vi "HostToFPGA(RGB).vi"(7 "Maximum Pixels per Write":i32=-1, 8 "error in (no error)":errorcluster, 9 "FPGA Reference in":refnum<k20>, 10 "Write Timeout (ms)":i32=5000, 11 "Image in":T1) -> (0 "error out":errorcluster, 3 "Image out":T1)   [LabVIEW 2016]
uses:
  <vilib>/vision/Image Controls.llb/IMAQ Image.ctl
  <vilib>/vision/EDVR.llb/IMAQ ImageToEDVR 2D U32.vi
  <vilib>/rvi/errors/niLvFpgaAdjustHostInterfaceError.vi
  <vilib>/rvi/interface/nirviMethod/nirviMethod.xnode
  <vilib>/FPGAPlugInAG/Dynamic/niLvFpga_WriteFifo_Dynamic.vi
  <vilib>/rvi/errors/niLvFpgaMergeErrorWithErrorCode.vi
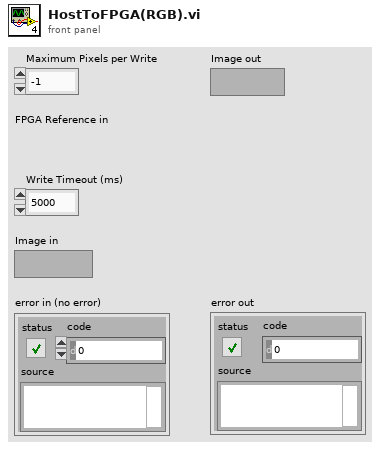
[diagram p1: front panel]
types:
  T1 = typedef "IMAQ Image.ctl" = refnum<image>
  T2 = typedef "Image Type" = u32
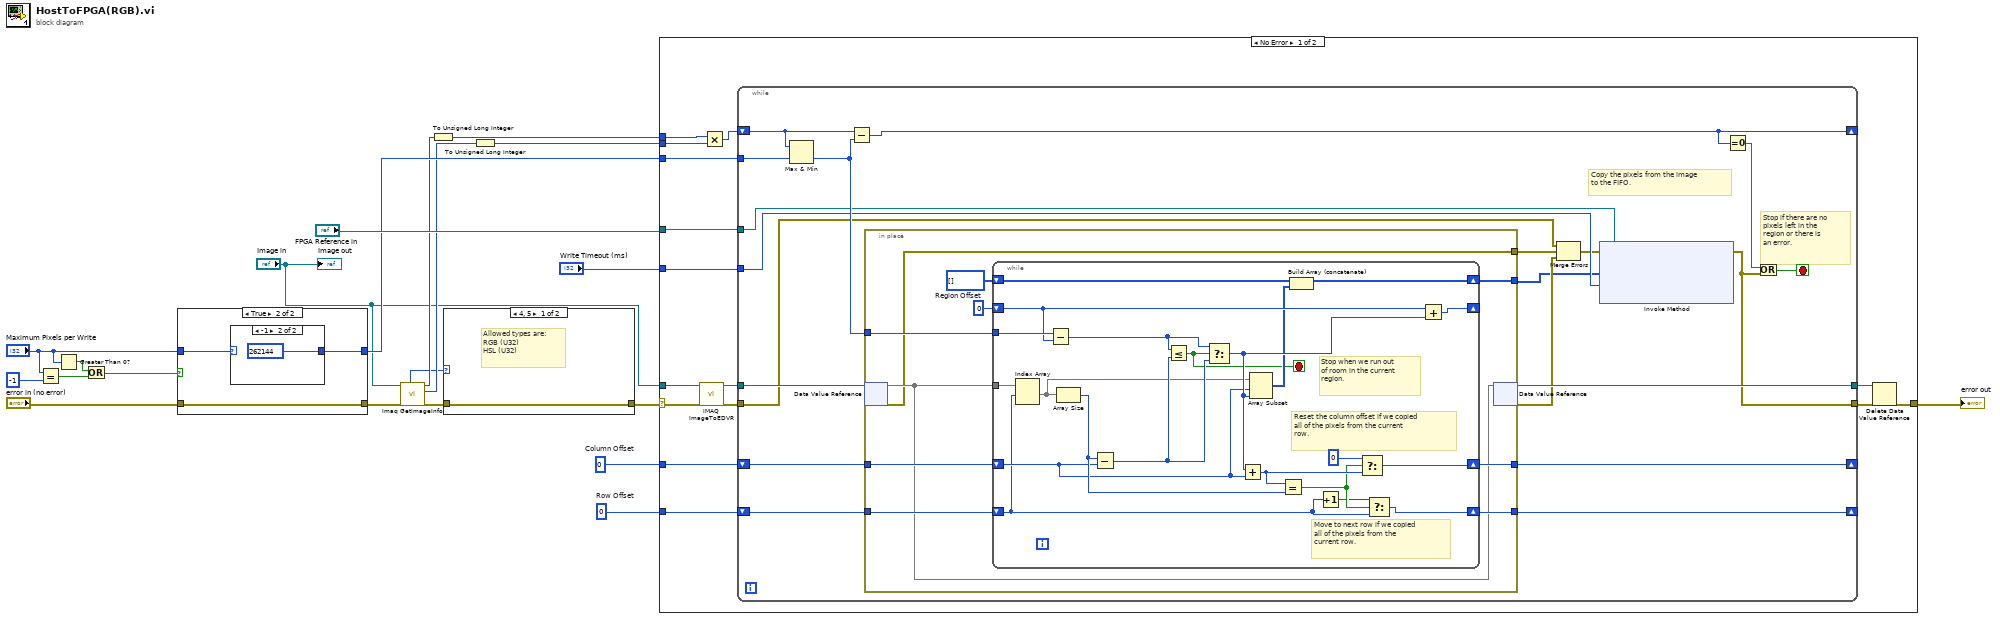
[diagram p0: block diagram]
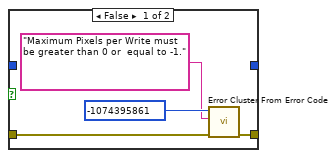
[diagram p2: hidden frame]
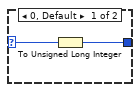
[diagram p3: hidden frame]
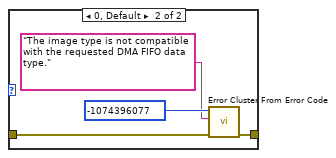
[diagram p4: hidden frame]
diagram:
  w14 = u32 0  # Row Offset
  w15 = u32 0  # Column Offset
  n1 = Equal?(x="Maximum Pixels per Write", y=-1) -> (x = y?=w5:bool)
  n2 = Greater Than 0?(x="Maximum Pixels per Write") -> (x > 0?=w4:bool)
  n3 = Or(x=w4, y=w5) -> (x .or. y?=w6:bool)
  n4 = case shown="True" w6 {
    tunnel: "error in (no error)" -> [w23 w28]
    tunnel: [w22 w28] -> w12
    tunnel: "Maximum Pixels per Write" -> [_ w27]
    tunnel: [_ w26] -> w18
    frame False {
      n5 = call <vilib>:"Error Cluster From Error Code.vi"("error in (no error)"=w23, "error message (\"\")"="Maximum Pixels per Write must be greater than 0 or  equal to -1." ("error message (\"\")"), "error code (0)"=-1074395861) -> ("error out"=w22:errorcluster)  [unwired: 6 in]
    }
    frame True {
      n6 = case shown="-1" w27 {
        selector: w27 -> [w30 _]
        tunnel: [w29 u32 262144 ("Maximum Pixels per Write")] -> w26
        frame 0, Default {
          n7 = To Unsigned Long Integer(number=w30) -> (unsigned 32bit integer=w29:u32)
        }
        frame -1 {
        }
      }
    }
  }
  n8 = call "Imaq GetImageInfo"("error in (no error)"=w12, "Image"="Image in") -> ("error out"=w11:errorcluster, "Y Resolution"=w17:i32, "X Resolution"=w13:i32, "Image Type"=w10:T2)  [unwired: 2 in, 4 out]
  n9 = To Unsigned Long Integer(number=w13) -> (unsigned 32bit integer=w19:u32)
  n10 = case shown="4, 5" w10 {
    tunnel: w11 -> [w32 w34]
    tunnel: [w32 w33] -> w16
    frame 4, 5 {
      # "Allowed types are:\nRGB (U32)\nHSL (U32)"
    }
    frame 0, Default {
      n11 = call <vilib>:"Error Cluster From Error Code.vi"("error in (no error)"=w34, "error message (\"\")"="The image type is not compatible with the requested DMA FIFO data type." ("error message (\"\")"), "error code (0)"=-1074396077) -> ("error out"=w33:errorcluster)  [unwired: 6 in]
    }
  }
  n12 = To Unsigned Long Integer(number=w17) -> (unsigned 32bit integer=w20:u32)
  n13 = case shown="No Error" w16 {
    selector: w16 -> [w46 w103]
    tunnel: w15 -> [w48 _]
    tunnel: w14 -> [w47 _]
    tunnel: "FPGA Reference in" -> [w50 _]
    tunnel: [w44 w103] -> w8
    tunnel: w18 -> [w51 _]
    tunnel: "Write Timeout (ms)" -> [w49 _]
    tunnel: "Image in" -> [w45 _]
    tunnel: w19 -> [w43 _]
    tunnel: w20 -> [w42 _]
    frame No Error {
      n14 = call-poly <vilib>:"IMAQ ImageToEDVR.vi"("error out"=w46, "Image"=w45) -> ("error out"=w40:errorcluster, "EDVR 2D U32"=w41:refnum<data-value>)  [unwired: 7 in, 1 out]
      n15 = Multiply(x=w43, y=w42) -> (x*y=w37:u32)
      n16 = while {
        shift-right: [w65] -> _
        shift-left: w37 -> [w62]
        tunnel: w41 -> [w71]
        shift-right: [w67] -> _
        shift-left: w48 -> [w69]
        shift-right: [w70] -> _
        shift-left: w47 -> [w68]
        tunnel: w50 -> [w56]
        tunnel: [w66] -> w39
        tunnel: [w54] -> w38
        tunnel: w51 -> [w61]
        tunnel: w49 -> [w57]
        tunnel: w40 -> [w52]
        stop <- w64 stop-if-true
        # "Copy the pixels from the image\nto the FIFO."
        # "Stop if there are no\npixels left in the \nregion or there is\nan error."
        n17 = Max & Min(x=w62, y=w61) -> (min(x,y)=w60:u32)  [unwired: 1 out]
        n18 = Subtract(x=w62, y=w60) -> (x-y=w65:u32)
        n19 = in-place {
          in-place-border: w60 -> [w79]
          in-place-border: [w81] -> w70
          in-place-border: w69 -> [w78]
          in-place-border: w68 -> [w76]
          in-place-border: [w77] -> w67
          in-place-border: [w73] -> w59
          in-place-border: [w72] -> w53
          w80 = u32 0  # Region Offset
          n20 = in-place-dvr #1(w71) -> (w75:u32[][], w73:errorcluster)
          n21 = while {
            tunnel: w75 -> [w88]
            shift-right: [w100] -> _
            shift-left: w80 -> [w99]
            tunnel: w79 -> [w102]
            shift-right: [w93] -> w77
            shift-left: w78 -> [w89]
            shift-right: [w83] -> w72
            shift-left: u8[] [] -> [w85]
            shift-right: [w90] -> w81
            shift-left: w76 -> [w86]
            stop <- w82 stop-if-true
            # "Stop when we run out\nof room in the current\nregion."
            # "Reset the column offset if we copied\nall of the pixels from the current\nrow."
            # "Move to next row if we copied\nall of the pixels from the\ncurrent row."
            n22 = Index Array(array=w88, index (row)=w86) -> (element=w87:u32[])  [unwired: 1 in]
            n23 = Subtract(x=w102, y=w99) -> (x-y=w101:u32)
            n24 = Array Size(array=w87) -> (size(s)=w98:i32)
            n25 = Subtract(x=w98, y=w89) -> (x-y=w96:u32)
            n26 = Less Or Equal?(x=w101, y=w96) -> (x <= y?=w82:bool)
            n27 = Select(t=w101, s=w82, f=w96) -> (s? t:f=w97:u32)
            n28 = Add(x=w97, y=w89) -> (x+y=w94:u32)
            n29 = Array Subset(array=w87, index=w89, length=w97) -> (w84:u32[])
            n30 = Equal?(x=w94, y=w98) -> (x = y?=w92:bool)
            n31 = Build Array (concatenate)(w85, w84) -> (w83:u32[])
            n32 = Increment(x=w86) -> (x+1=w91:u32)
            n33 = Select(t=u32 0 ("Elements In Region"), s=w92, f=w94) -> (s? t:f=w93:u32)
            n34 = Select(t=w91, s=w92, f=w86) -> (s? t:f=w90:u32)
            n35 = Add(x=w99, y=w97) -> (x+y=w100:u32)
          }
          n36 = in-place-dvr #1(w75) -> (w66:refnum<data-value>, w58:errorcluster)
        }
        n37 = Merge Errors(w52, w59, w58) -> (w55:errorcluster)
        n38 = xnode "Invoke Method"("FPGA VI Reference In"=w56, "error in"=w55, "Data"=w53, "Timeout (ms)"=w57) -> ("error out"=w54:errorcluster)  [unwired: 2 out]
        n39 = Equal To 0?(x=w65) -> (x = 0?=w63:bool)
        n40 = Or(x=w63, y=w54) -> (x .or. y?=w64:bool)
      }
      n41 = Delete Data Value Reference(data value reference=w39, error in=w38) -> (error out=w44:errorcluster)  [unwired: 1 out]
    }
    frame Error {
    }
  }
  "error out" <- w8
  "Image out" <- "Image in"
